vi "SSH_cmds.vi"(7 "Commands":string[](array[string]), 8 "error in (no error)":errorcluster, 10 "Console In":string, 11 "Python in":cluster{"Python":refnum<k35>, "py file":path}) -> (0 "error out":errorcluster, 2 "Console Out":string, 3 "Python out":cluster{"Python":refnum<k35>, "py file":path})   [LabVIEW 2020]
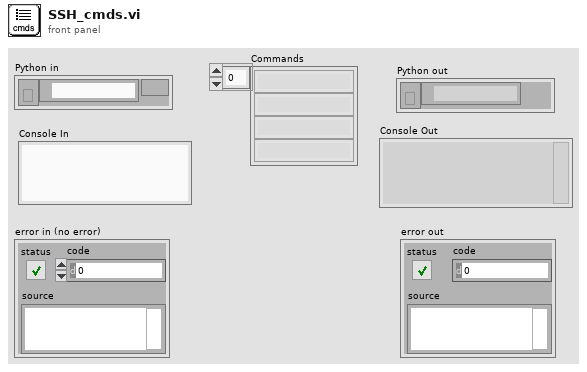
[diagram p1: front panel]
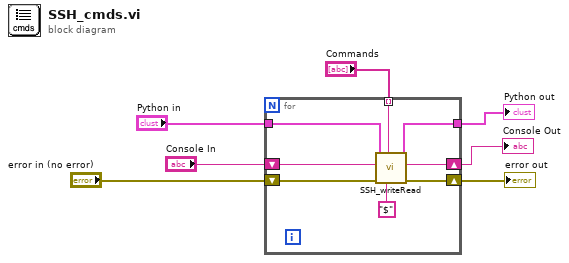
[diagram p0: block diagram]
diagram:
  n1 = for {
    tunnel: "Commands" -> [w12] mode=indexing
    shift-right: [w10] -> w5
    shift-left: "Console In" -> [w15]
    shift-right: [w9] -> w7
    shift-left: "error in (no error)" -> [w13]
    tunnel: "Python in" -> [w14]
    tunnel: [w8] -> w1
    n2 = call "SSH_writeRead.vi"("EOL"="$" ("function name"), "Text"=w12, "error in (no error)"=w13, "Console In"=w15, "Python in"=w14) -> ("error out"=w9:errorcluster, "Console Out"=w10:string, "Python out"=w8:cluster{"Python":refnum<k35>, "py file":path})  [unwired: 4 in]
  }
  "Python out" <- w1
  "error out" <- w7
  "Console Out" <- w5
